vi "FTW-ActorContext-GetActorContext.vi"(8 "error in":errorcluster, 11 "Actor Context":refnum<class "FTW-Actor-Context.lvclass">) -> (0 "error out":errorcluster, 2 "Use Local Context":bool, 3 "Actor Context":refnum<vi>)   [LabVIEW 2014, in "FTW-Actor-Context.lvclass"]
uses:
  FTW-Actor-Context.lvclass
panel:
  # "Inputs"
  # "Outputs"
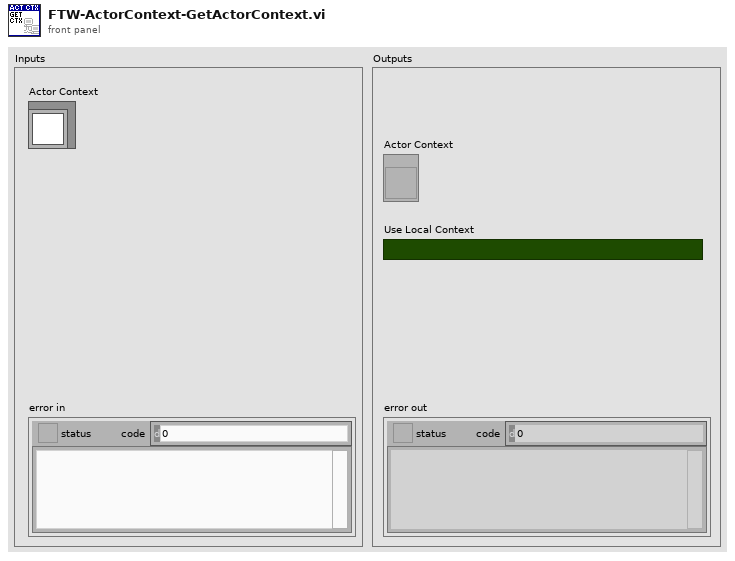
[diagram p1: front panel]
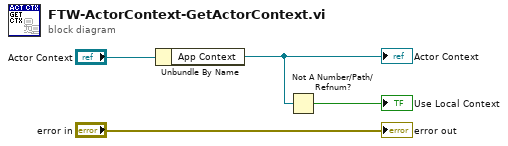
[diagram p0: block diagram]
diagram:
  n1 = Unbundle By Name("Actor Context") -> ("App Context"=w2:refnum<vi>)
  "Actor Context" <- w2
  n2 = Not A Number/Path/Refnum?(number/path/refnum=w2) -> (NaN/Path/Refnum?=→"Use Local Context":bool)
  "error out" <- "error in"
